vi "PFI-28000-Card_Create.vi"(0 "PFI-28000-Card in":refnum<class "PFI-28000-Card.lvclass">, 5 "Card Info":T1, 7 "System":refnum<class "PFI-28000-System.lvclass">, 11 "error in (no error)":errorcluster) -> (4 "PFI-28000-Card out":refnum<class "PFI-28000-Card.lvclass">, 15 "error out":errorcluster)   [LabVIEW 2017, in "PFI-28000-Card.lvclass"]
uses:
  PFI-28000-Card.lvclass
  PFI-28000-Card-Card Info.ctl
  System/PFI-28000-System.lvclass
  C:/wc/07143 Precision Filters 28000 Support/Driver/source/Base/PFI-28000-Base.lvclass
  PFI-28000-Card.lvclass/PFI-28000-Card.ctl
  Channel/PFI-28000-Channel.lvclass
  28144 Channel/PFI-28000-Chan-28144.lvclass
  C:/wc/07143 Precision Filters 28000 Support/Driver/source/Channel/PFI-28000-Channel.lvclass
  Utilities/PFI-28000-Utils.lvlib
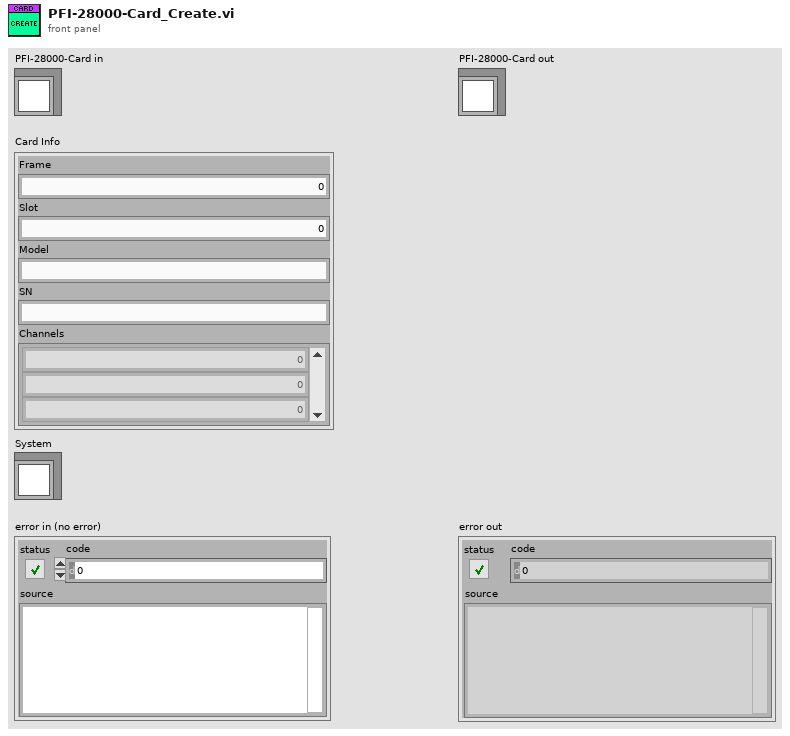
[diagram p1: front panel]
types:
  T1 = typedef "PFI-28000-Card.lvclass/PFI-28000-Card-Card Info.ctl" = cluster{"Frame":i32, "Slot":i32, "Model":string, "SN":string, "Channels":i32[]}
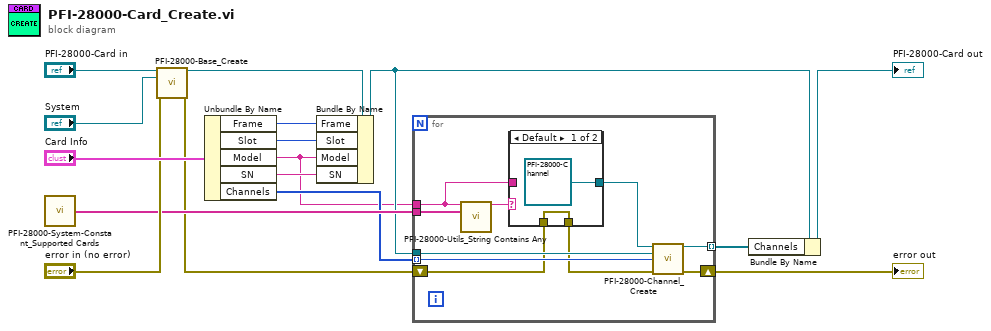
[diagram p0: block diagram]
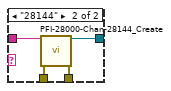
[diagram p2: hidden frame]
diagram:
  n1 = call "PFI-28000-System-Constant_Supported Cards.vi"() -> ("Supported Cards"=w8:string[])  [unwired: 15 in]
  n2 = call-dynamic "PFI-28000-Base_Create.vi"("PFI-28000-Base in"="PFI-28000-Card in", "Parent"="System", "error in (no error)"="error in (no error)") -> ("PFI-28000-Base out"=w11:refnum<class "PFI-28000-Card.lvclass">, "error out"=w6:errorcluster)  [unwired: 11 in]
  n3 = Unbundle By Name("Card Info") -> ("Frame"=w15:i32, "Slot"=w14:i32, "Model"=w1:string, "SN"=w13:string, "Channels"=w7:i32[])
  n4 = Bundle By Name(cluster=w11, "Frame"=w15, "Slot"=w14, "Model"=w1, "SN"=w13) -> (w4:refnum<class "PFI-28000-Card.lvclass">)
  n5 = for {
    tunnel: w8 -> [w26]
    tunnel: w4 -> [w23]
    tunnel: w7 -> [w22] mode=indexing
    shift-right: [w21] -> w5
    shift-left: w6 -> [w18]
    tunnel: [w20] -> w2 mode=indexing
    tunnel: w1 -> [w19]
    n6 = call "PFI-28000-Utils_String Contains Any.vi"("String"=w19, "Values"=w26) -> ("Match"=w25:string)  [unwired: 11 in, 2 out]
    n7 = case shown="Default" w25 {
      tunnel: [refnum<class "PFI-28000-Channel.lvclass"> refnum ("PFI-28000-Channel") w32] -> w24
      tunnel: w19 -> [_ w31]
      tunnel: w18 -> [w27 w30]
      tunnel: [w27 w29] -> w17
      frame Default {
      }
      frame "28144" {
        n8 = call "PFI-28000-Chan-28144_Create.vi"("Model String"=w31, "error in (no error)"=w30) -> ("PFI-28000-Chan-28144 out"=w32:refnum<class "PFI-28000-Chan-28144.lvclass">, "error out"=w29:errorcluster)  [unwired: 12 in]
      }
    }
    n9 = call-dynamic "PFI-28000-Channel_Create.vi"("PFI-28000-Channel in"=w24, "Parent"=w23, "Channel Number"=w22, "error in (no error)"=w17) -> ("PFI-28000-Channel out"=w20:refnum<class "PFI-28000-Channel.lvclass">, "error out"=w21:errorcluster)  [unwired: 10 in]
  }
  "error out" <- w5
  n10 = Bundle By Name(cluster=w4, "Channels"=w2) -> (→"PFI-28000-Card out":refnum<class "PFI-28000-Card.lvclass">)
